vi "RT.vi"() -> ()   [LabVIEW 2014]
uses:
  support/Message Queue/Kapitza Message Queue.lvlib
  support/User Event - Stop/Kapitza User Event - Stop.lvlib
  support/Message Queue/Enqueue Message (Single).vi
  Classes/Abstract/Data/Data2D/Data2D.lvclass
  Classes/Abstract/Measurement/Measurement2D/Measurement2D.lvclass
  Classes/2D/RT/RT.lvclass
panel:
  in  "File Path Control":path=path "C:/Users/Sergei/Documents"
  in  "Driver 1":path=path "C:/Users/Sergei/YandexDisk/Лаборатория/Projects/Kapitza_prealpha/Drivers/Simulator.vi"
  in  "Driver 2":path=path "C:/Users/Sergei/YandexDisk/Лаборатория/Projects/Kapitza_prealpha/Drivers/Simulator.vi"
  in  "Address 2":refnum<visa-resource-name>
  in  "Address 1":refnum<visa-resource-name>
  in  "Stop":bool
  in  "Sample Name":string
  in  "Max":dbl
  in  "Step":dbl
  in  "Init":dbl
  in  "x0,5 step":bool
  out "y":dbl
  out "x":dbl
  in  "x2 step":bool
  in  "Start":bool
  out "XY Graph":cluster{"X":dbl[], "Y":dbl[]}[](graph)
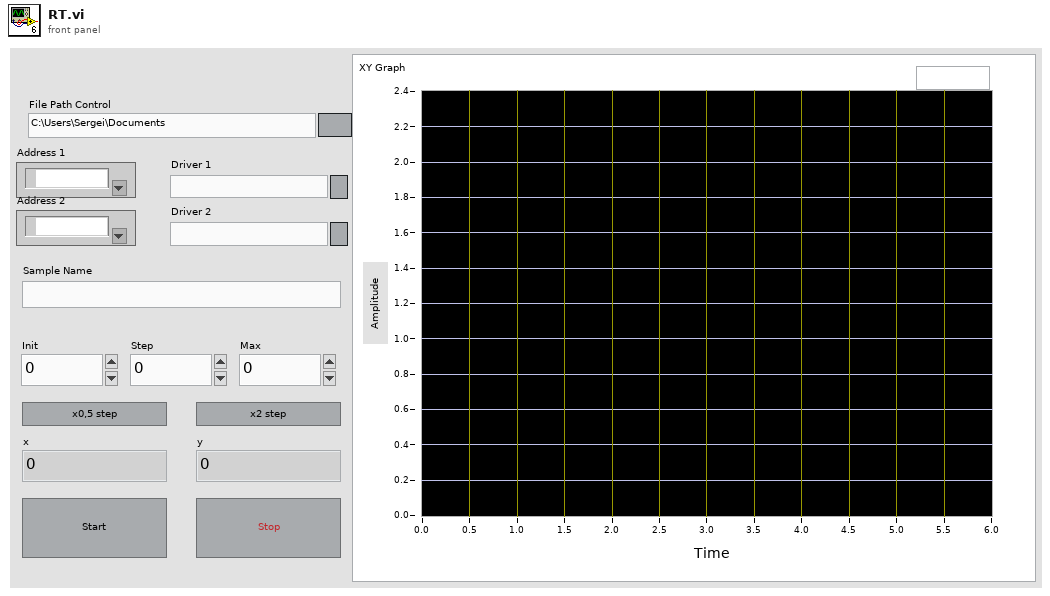
[diagram p1: front panel]
types:
  T1 = typedef "Kapitza Message Queue.lvlib/All Message Queues.ctl" = cluster{"UI":refnum<queue>}
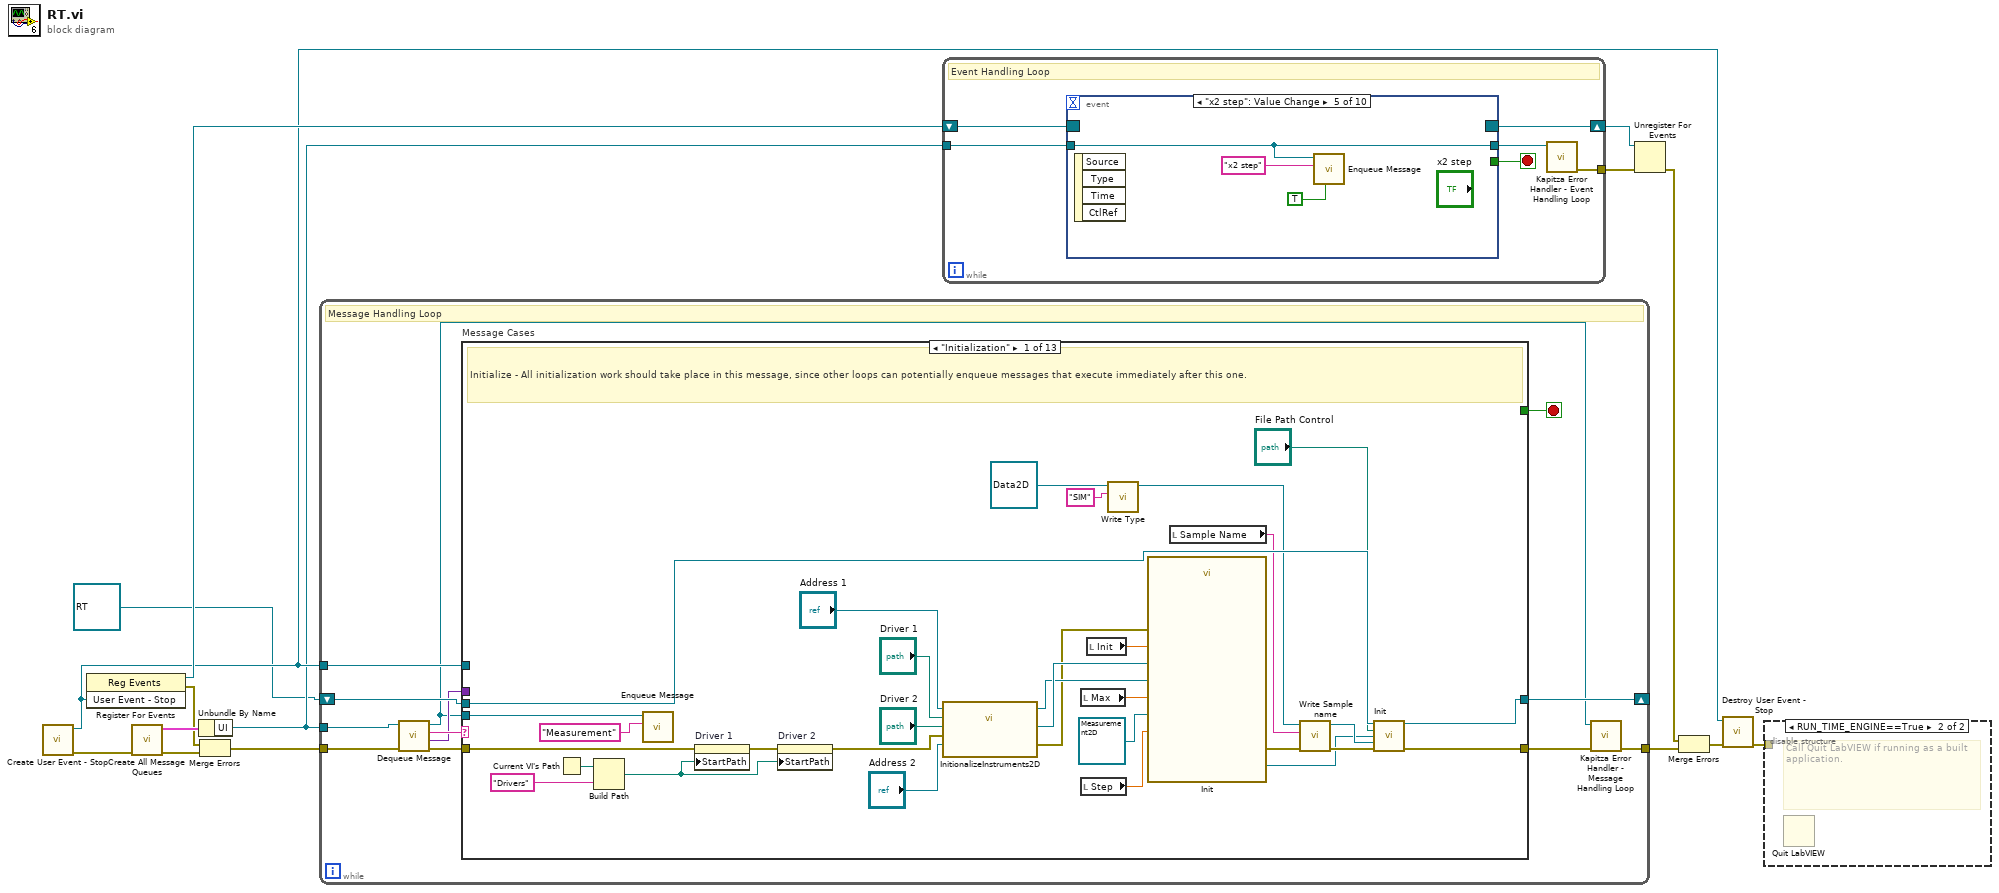
[diagram p0: block diagram]
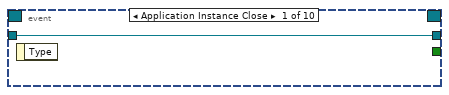
[diagram p3: hidden frame]
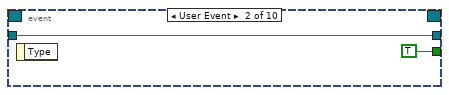
[diagram p4: hidden frame]
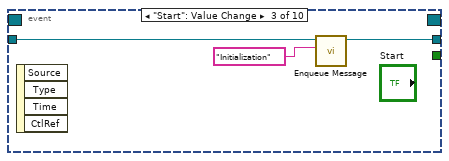
[diagram p5: hidden frame]
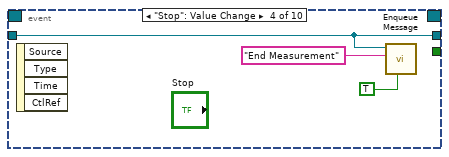
[diagram p6: hidden frame]
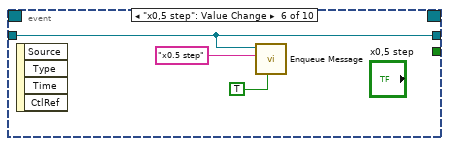
[diagram p7: hidden frame]
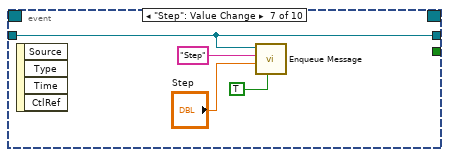
[diagram p8: hidden frame]
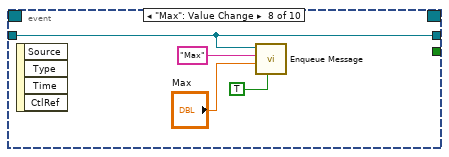
[diagram p9: hidden frame]
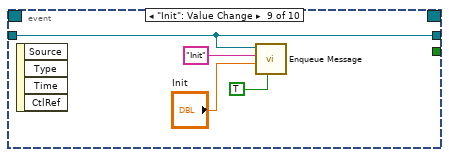
[diagram p10: hidden frame]
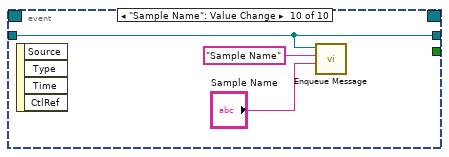
[diagram p11: hidden frame]
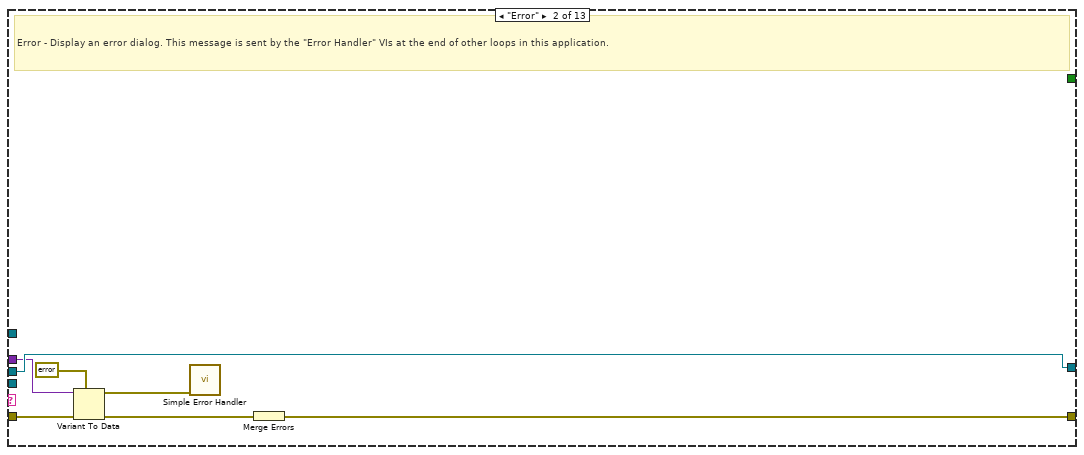
[diagram p12: hidden frame]
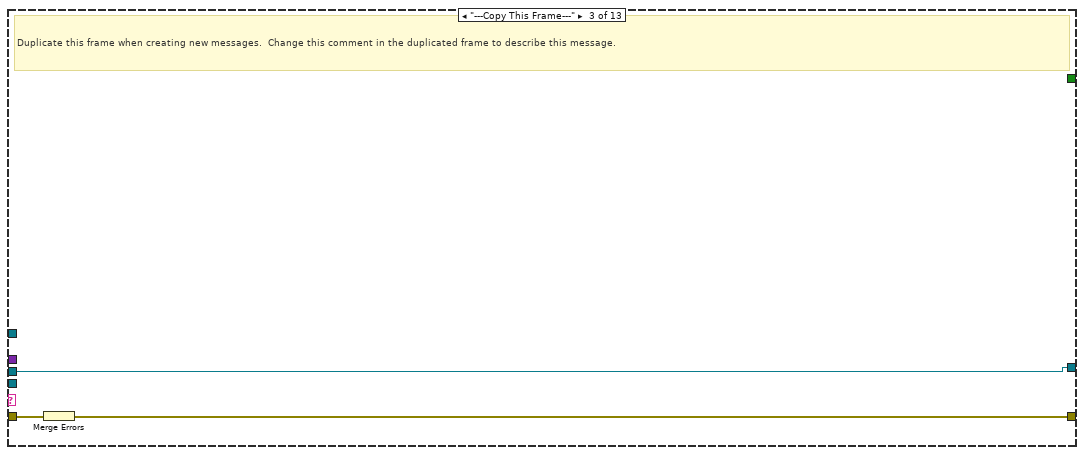
[diagram p13: hidden frame]
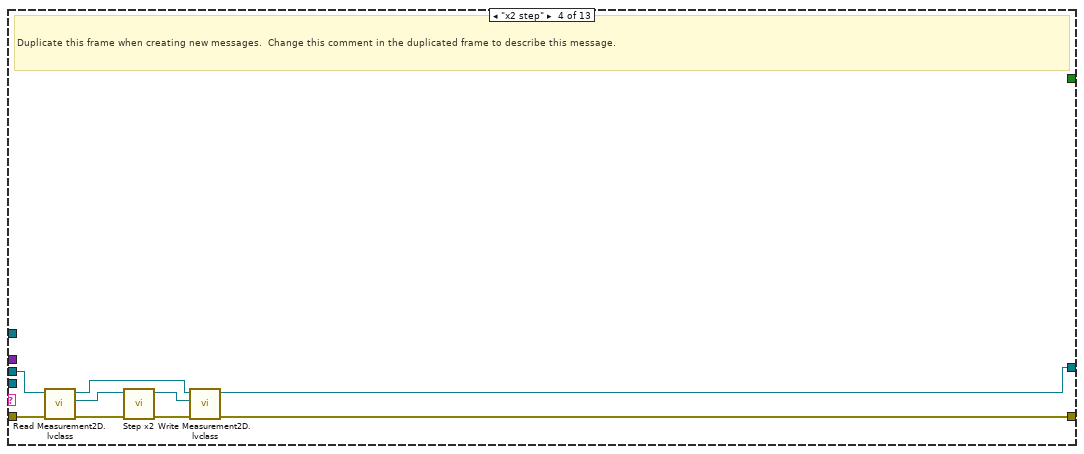
[diagram p14: hidden frame]
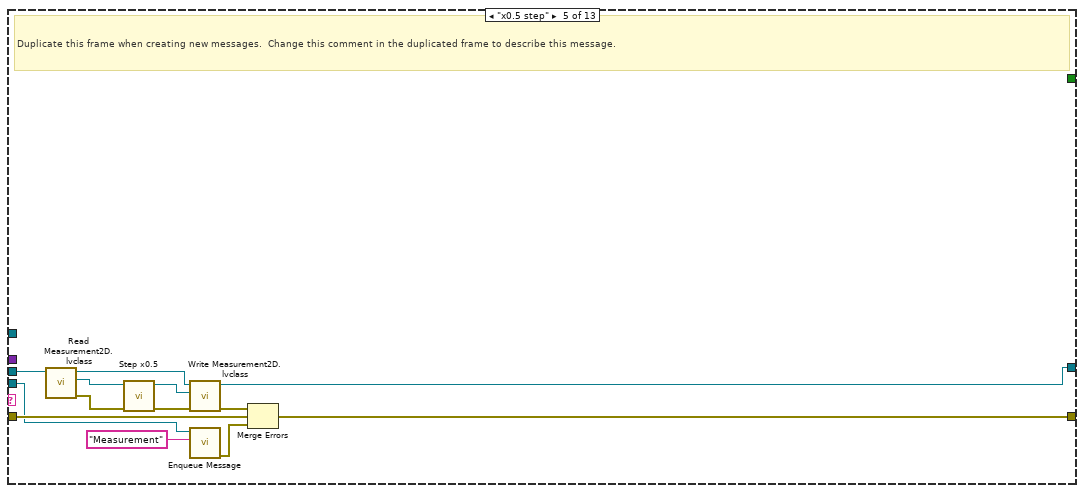
[diagram p15: hidden frame]
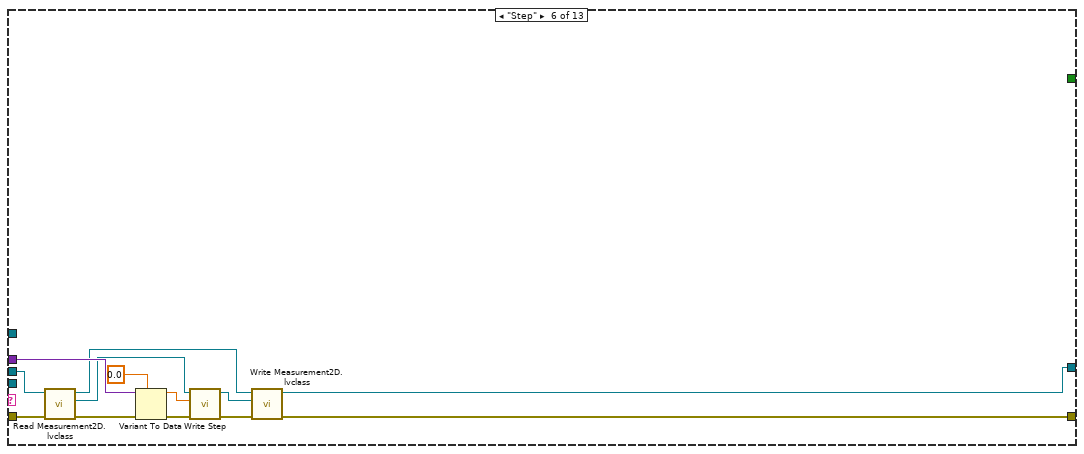
[diagram p16: hidden frame]
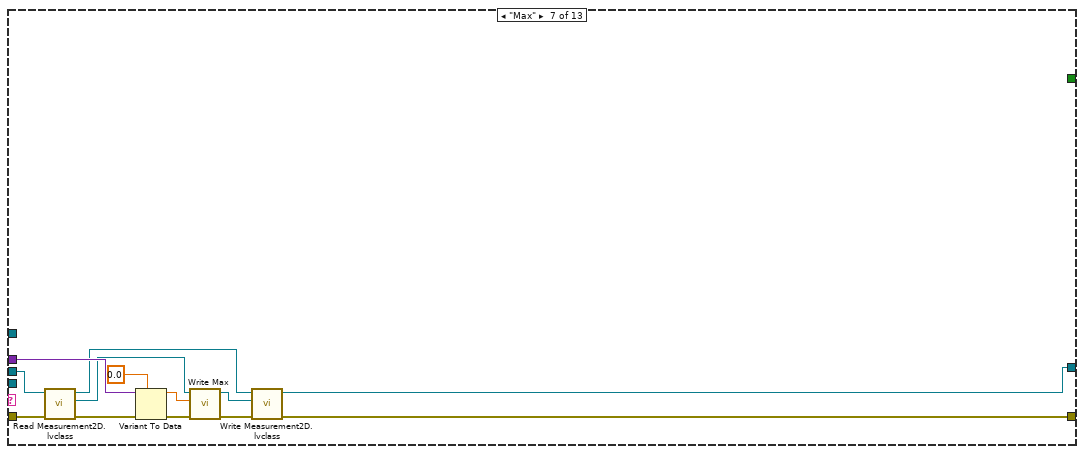
[diagram p17: hidden frame]
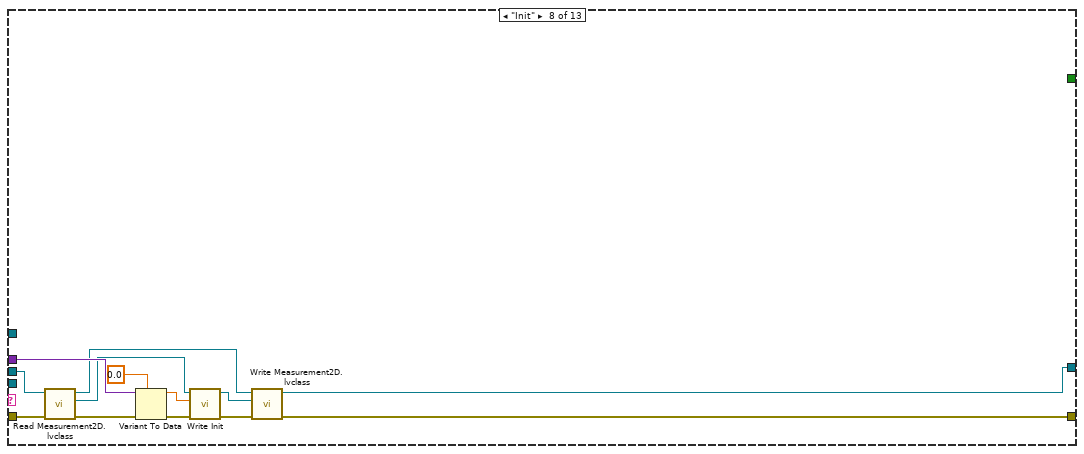
[diagram p18: hidden frame]
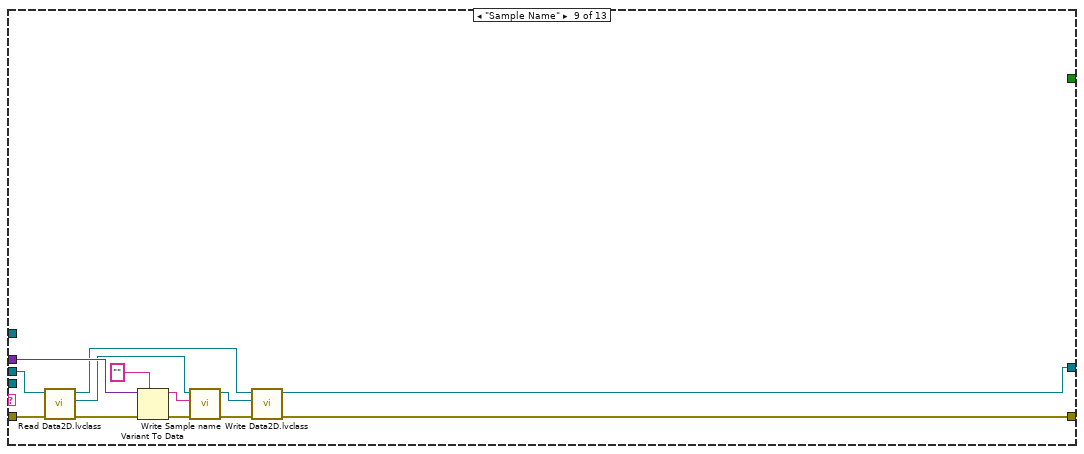
[diagram p19: hidden frame]
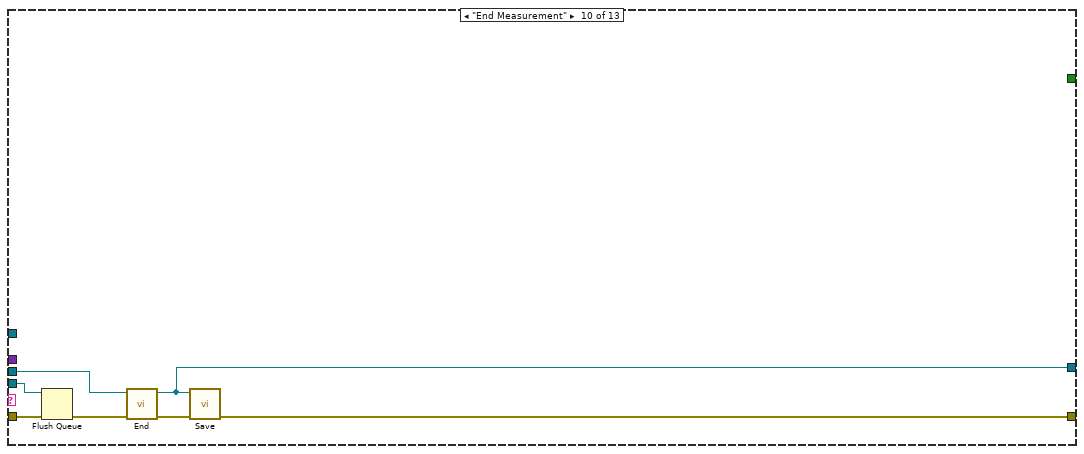
[diagram p20: hidden frame]
diagram:
  n1 = call "Create User Event - Stop.vi"() -> ("error out"=w13:errorcluster, "User Event - Stop"=w6:refnum<user-event>)  [unwired: 10 in]
  n2 = register-events(w6) -> (reference out=w7:refnum<event-registration>, error out=w4:errorcluster)  [unwired: 2 in]
  n3 = call "Create All Message Queues.vi"("error in (no error)"=w13) -> ("error out"=w2:errorcluster, "Message Queues out"=w15:T1)  [unwired: 9 in]
  n4 = Unbundle By Name(w15) -> ("UI"=w3:refnum<queue>)
  n5 = Merge Errors(w4, w2) -> (w5:errorcluster)
  n6 = while {
    tunnel: w3 -> [w19]
    shift-right: [w26] -> _
    shift-left: refnum<class "RT.lvclass"> refnum ("RT.lvclass") -> [w27]
    tunnel: w6 -> [w24]
    tunnel: w5 -> [w23]
    tunnel: [w17] -> w14
    stop <- w25 stop-if-true
    # "Message Handling Loop"
    n7 = call "Dequeue Message.vi"("error in (no error)"=w23, "Message Queue"=w19) -> ("error out"=w22:errorcluster, "Message Data"=w20:variant, "Message"=w21:string, "dup Message Queue"=w18:refnum<queue>)  [unwired: 6 in]
    n8 = case "Message Cases" shown="\"Initialization\"" w21 {
      tunnel: w18 -> [w33 _ _ _ w83 _ _ _ _ w147 w166 w187 _]
      tunnel: w22 -> [w38 w65 w68 w70 w90 w94 w108 w121 w134 w145 w151 w180 w188]
      tunnel: [w28 w59 w66 w69 w89 w91 w104 w117 w130 w143 w165 w183 w188] -> w16
      tunnel: w27 -> [w58 w64 w67 w77 w88 w100 w110 w126 w140 w149 w168 w186 w189]
      tunnel: [w57 w64 w67 w73 w86 w99 w109 w125 w139 w148 w157 w186 w189] -> w26
      tunnel: [_ _ _ _ _ _ _ _ _ _ _ TRUE _] -> w25
      tunnel: w20 -> [_ w63 _ _ _ w103 w116 w129 w142 _ _ w177 _]
      tunnel: w24 -> [_ _ _ _ _ _ _ _ _ _ _ w182 _]
      frame "Initialization" {
        # "Initialize - All initialization work should take place in this message, since other loops can potentially enqueue messages that execute immediately after this one."
        n9 = Current VI's Path() -> (path=w40:path)
        n10 = Build Path(base path=w40, name or relative path="Drivers") -> (appended path=w36:path)
        n11 = call-poly "Enqueue Message.vi"("Message"="Measurement", "Message Queue"=w33) -> ()  [unwired: 8 in, 2 out]
        n12 = property on="Driver 1" class="Path"(error in=w38, "StartPath"=w36) -> (error out=w37:errorcluster)  [unwired: 1 in, 1 out]
        n13 = property on="Driver 2" class="Path"(error in=w37, "StartPath"=w36) -> (error out=w35:errorcluster)  [unwired: 1 in, 1 out]
        n14 = call "InitionalizeInstruments2D.vi"("Address in"="Address 2", "error in (no error)"=w35, "Driver in"="Driver 2", "Driver 1"="Driver 1", "VISA Refnum in"="Address 1") -> ("error out"=w45:errorcluster, "Instrument out 2"=w52:refnum<class "Instrument.lvclass">, "Instrument out"=w51:refnum<class "Instrument.lvclass">)  [unwired: 4 in]
        n15 = local read "Max"() -> (w50:dbl)
        n16 = local read "Step"() -> (w49:dbl)
        n17 = local read "Init"() -> (w48:dbl)
        n18 = call-dynamic "Write Type.vi"("Type"="SIM", "Data2D in"=refnum<class "Data2D.lvclass"> refnum ("Data2D.lvclass")) -> ("Data2D out"=w30:refnum<class "Data2D.lvclass">)  [unwired: 8 in, 1 out]
        n19 = call-dynamic "Init.vi"("Instrument.lvclass 2"=w51, "Step"=w49, "Instrument 1.lvclass"=w52, "error in (no error)"=w45, "Max"=w50, "Init"=w48, "Measurement1D in"=refnum<class "Measurement2D.lvclass"> refnum) -> ("error out"=w44:errorcluster, "Measurement1D out"=w41:refnum<class "Measurement2D.lvclass">)  [unwired: 3 in]
        n20 = local read "Sample Name"() -> (w46:string)
        n21 = call-dynamic "Write Sample name.vi"("error in (no error)"=w44, "Sample name"=w46, "Data2D in"=w30) -> ("error out"=w43:errorcluster, "Data2D out"=w42:refnum<class "Data2D.lvclass">)  [unwired: 7 in]
        n22 = call-dynamic "Init.vi"("Experiment2D in"=w58, "Path"="File Path Control", "Measurement2D.lvclass"=w41, "Data2D.lvclass"=w42, "error in (no error)"=w43) -> ("Experiment2D out"=w57:refnum<class "RT.lvclass">, "error out"=w28:errorcluster)  [unwired: 9 in]
      }
      frame "Error" {
        # "Error - Display an error dialog. This message is sent by the \"Error Handler\" VIs at the end of other loops in this application."
        n23 = Variant To Data(error in=w65, type=errorcluster {"status"=FALSE, "code"=0, "source"=""} ("error constant"), Variant=w63) -> (data=w61:errorcluster, error out=w60:errorcluster)
        n24 = call <vilib>:"Simple Error Handler.vi"("error in (no error)"=w61) -> ()  [unwired: 4 in, 5 out]
        n25 = Merge Errors(w60) -> (w59:errorcluster)
      }
      frame "---Copy This Frame---" {
        # "Duplicate this frame when creating new messages.  Change this comment in the duplicated frame to describe this message."
        n26 = Merge Errors(w68) -> (w66:errorcluster)
      }
      frame "x2 step" {
        # "Duplicate this frame when creating new messages.  Change this comment in the duplicated frame to describe this message."
        n27 = call-dynamic "Read Measurement2D.lvclass.vi"("error in (no error)"=w70, "Experiment2D in"=w77) -> ("error out"=w72:errorcluster, "Measurement2D.lvclass"=w76:refnum<class "Measurement2D.lvclass">, "Experiment2D out"=w75:refnum<class "RT.lvclass">)  [unwired: 7 in]
        n28 = call-dynamic "Step x2.vi"("error in (no error)"=w72, "Measurement2D in"=w76) -> ("error out"=w71:errorcluster, "Measurement2D out"=w74:refnum<class "Measurement2D.lvclass">)  [unwired: 8 in]
        n29 = call-dynamic "Write Measurement2D.lvclass.vi"("error in (no error)"=w71, "Measurement2D.lvclass"=w74, "Experiment2D in"=w75) -> ("error out"=w69:errorcluster, "Experiment2D out"=w73:refnum<class "RT.lvclass">)  [unwired: 7 in]
      }
      frame "x0.5 step" {
        # "Duplicate this frame when creating new messages.  Change this comment in the duplicated frame to describe this message."
        n30 = call-dynamic "Read Measurement2D.lvclass.vi"("Experiment2D in"=w88) -> ("error out"=w78:errorcluster, "Measurement2D.lvclass"=w85:refnum<class "Measurement2D.lvclass">, "Experiment2D out"=w87:refnum<class "RT.lvclass">)  [unwired: 8 in]
        n31 = call-dynamic "Step x0.5.vi"("error in (no error)"=w78, "Measurement2D in"=w85) -> ("error out"=w79:errorcluster, "Measurement2D out"=w84:refnum<class "Measurement2D.lvclass">)  [unwired: 8 in]
        n32 = call-dynamic "Write Measurement2D.lvclass.vi"("error in (no error)"=w79, "Measurement2D.lvclass"=w84, "Experiment2D in"=w87) -> ("error out"=w81:errorcluster, "Experiment2D out"=w86:refnum<class "RT.lvclass">)  [unwired: 7 in]
        n33 = call-poly "Enqueue Message.vi"("Message"="Measurement", "Message Queue"=w83) -> ("error out"=w80:errorcluster)  [unwired: 8 in, 1 out]
        n34 = Merge Errors(w81, w90, w80) -> (w89:errorcluster)
      }
      frame "Step" {
        n35 = call-dynamic "Read Measurement2D.lvclass.vi"("error in (no error)"=w94, "Experiment2D in"=w100) -> ("error out"=w93:errorcluster, "Measurement2D.lvclass"=w98:refnum<class "Measurement2D.lvclass">, "Experiment2D out"=w101:refnum<class "RT.lvclass">)  [unwired: 7 in]
        n36 = Variant To Data(error in=w93, type=0.0, Variant=w103) -> (data=w97:dbl, error out=w92:errorcluster)
        n37 = call-dynamic "Write Step.vi"("error in (no error)"=w92, "Step"=w97, "Measurement2D in"=w98) -> ("error out"=w95:errorcluster, "Measurement2D out"=w96:refnum<class "Measurement2D.lvclass">)  [unwired: 7 in]
        n38 = call-dynamic "Write Measurement2D.lvclass.vi"("error in (no error)"=w95, "Measurement2D.lvclass"=w96, "Experiment2D in"=w101) -> ("error out"=w91:errorcluster, "Experiment2D out"=w99:refnum<class "RT.lvclass">)  [unwired: 7 in]
      }
      frame "Max" {
        n39 = call-dynamic "Read Measurement2D.lvclass.vi"("error in (no error)"=w108, "Experiment2D in"=w110) -> ("error out"=w107:errorcluster, "Measurement2D.lvclass"=w113:refnum<class "Measurement2D.lvclass">, "Experiment2D out"=w111:refnum<class "RT.lvclass">)  [unwired: 7 in]
        n40 = Variant To Data(error in=w107, type=0.0, Variant=w116) -> (data=w114:dbl, error out=w106:errorcluster)
        n41 = call-dynamic "Write Max.vi"("error in (no error)"=w106, "Max"=w114, "Measurement2D in"=w113) -> ("error out"=w105:errorcluster, "Measurement2D out"=w112:refnum<class "Measurement2D.lvclass">)  [unwired: 7 in]
        n42 = call-dynamic "Write Measurement2D.lvclass.vi"("error in (no error)"=w105, "Measurement2D.lvclass"=w112, "Experiment2D in"=w111) -> ("error out"=w104:errorcluster, "Experiment2D out"=w109:refnum<class "RT.lvclass">)  [unwired: 7 in]
      }
      frame "Init" {
        n43 = call-dynamic "Read Measurement2D.lvclass.vi"("error in (no error)"=w121, "Experiment2D in"=w126) -> ("error out"=w120:errorcluster, "Measurement2D.lvclass"=w124:refnum<class "Measurement2D.lvclass">, "Experiment2D out"=w127:refnum<class "RT.lvclass">)  [unwired: 7 in]
        n44 = Variant To Data(error in=w120, type=0.0, Variant=w129) -> (data=w123:dbl, error out=w119:errorcluster)
        n45 = call-dynamic "Write Init.vi"("error in (no error)"=w119, "Init"=w123, "Measurement2D in"=w124) -> ("error out"=w118:errorcluster, "Measurement2D out"=w122:refnum<class "Measurement2D.lvclass">)  [unwired: 7 in]
        n46 = call-dynamic "Write Measurement2D.lvclass.vi"("error in (no error)"=w118, "Measurement2D.lvclass"=w122, "Experiment2D in"=w127) -> ("error out"=w117:errorcluster, "Experiment2D out"=w125:refnum<class "RT.lvclass">)  [unwired: 7 in]
      }
      frame "Sample Name" {
        n47 = call-dynamic "Read Data2D.lvclass.vi"("error in (no error)"=w134, "Experiment2D in"=w140) -> ("error out"=w133:errorcluster, "Data2D.lvclass"=w137:refnum<class "Data2D.lvclass">, "Experiment2D out"=w135:refnum<class "RT.lvclass">)  [unwired: 7 in]
        n48 = Variant To Data(error in=w133, type="", Variant=w142) -> (data=w138:string, error out=w132:errorcluster)
        n49 = call-dynamic "Write Sample name.vi"("error in (no error)"=w132, "Sample name"=w138, "Data2D in"=w137) -> ("error out"=w131:errorcluster, "Data2D out"=w136:refnum<class "Data2D.lvclass">)  [unwired: 7 in]
        n50 = call-dynamic "Write Data2D.lvclass.vi"("error in (no error)"=w131, "Data2D.lvclass"=w136, "Experiment2D in"=w135) -> ("error out"=w130:errorcluster, "Experiment2D out"=w139:refnum<class "RT.lvclass">)  [unwired: 7 in]
      }
      frame "End Measurement" {
        n51 = Flush Queue(queue=w147, error in (no error)=w145) -> (error out=w144:errorcluster)  [unwired: 2 out]
        n52 = call-dynamic "End.vi"("error in (no error)"=w144, "Experiment2D in"=w149) -> ("error out"=w146:errorcluster, "Experiment2D out"=w148:refnum<class "RT.lvclass">)  [unwired: 8 in]
        n53 = call-dynamic "Save.vi"("error in (no error)"=w146, "Experiment2D in"=w148) -> ("error out"=w143:errorcluster)  [unwired: 8 in, 1 out]
      }
      frame "Measurement" {
        # "Duplicate this frame when creating new messages.  Change this comment in the duplicated frame to describe this message."
        n54 = call-dynamic "Measurement.vi"("error in (no error)"=w151, "Experiment2D in"=w168) -> ("error out"=w152:errorcluster, "Finish?"=w167:bool, "Experiment2D out"=w164:refnum<class "RT.lvclass">)  [unwired: 6 in, 1 out]
        n55 = Wait (ms)(milliseconds to wait=u32 100) -> ()  [unwired: 1 out]
        n56 = call-dynamic "Graph.vi"("error in (no error)"=w152, "Experiment2D in"=w164) -> ("error out"=w153:errorcluster, "Y"=w158:dbl[], "X"=w159:dbl[], "Experiment2D out"=w157:refnum<class "RT.lvclass">)  [unwired: 6 in]
        n57 = call-dynamic "Get point.vi"("error in (no error)"=w153, "Experiment2D in"=w157) -> ("error out"=w154:errorcluster, "y"=→"y":dbl, "x"=→"x":dbl)  [unwired: 6 in, 1 out]
        n58 = call "Convert to Dynamic Data"("Array"=w159) -> ("Dynamic Data Type"=w162:dynamicdata)  [unwired: 3 in]
        n59 = call "Convert to Dynamic Data2"("Array"=w158) -> ("Dynamic Data Type"=w161:dynamicdata)  [unwired: 3 in]
        n60 = call "Build XY Graph"("error in (no error)"=w154, "Y Input"=w161, "X Input"=w162) -> ("error out"=w150:errorcluster, "XY Graph"=→"XY Graph":cluster{"X":dbl[], "Y":dbl[]}[])  [unwired: 7 in]
        n61 = case shown="False" w167 {
          tunnel: w166 -> [w171 w176]
          tunnel: w150 -> [w170 w174]
          tunnel: [w169 w173] -> w165
          frame False {
            n62 = call-poly "Enqueue Message.vi"("error in (no error)"=w170, "Message"="Measurement", "Message Queue"=w171) -> ("error out"=w169:errorcluster)  [unwired: 7 in, 1 out]
          }
          frame True {
            n63 = call-poly "Enqueue Message.vi"("error in (no error)"=w174, "Message"="End Measurement", "Message Queue"=w176) -> ("error out"=w173:errorcluster)  [unwired: 7 in, 1 out]
          }
        }
      }
      frame "Exit" {
        # "Exit - Exit the application."
        n64 = Release Queue(queue=w187, error in (no error)=w180) -> (error out=w184:errorcluster)  [unwired: 1 in, 2 out]
        n65 = call "Fire User Event - Stop.vi"("User Event - Stop"=w182) -> ("error out"=w181:errorcluster)  [unwired: 10 in]
        n66 = Variant To Data(type=errorcluster {"status"=FALSE, "code"=0, "source"=""} ("error constant"), Variant=w177) -> (data=w178:errorcluster)  [unwired: 1 in, 1 out]
        n67 = Merge Errors(w181, w184) -> (w183:errorcluster)
        n68 = call <vilib>:"Simple Error Handler.vi"("error in (no error)"=w178) -> ()  [unwired: 4 in, 5 out]
      }
      frame Default {
        # "'Default' case only runs if there is a message that isn't defined in any of the other cases"
      }
    }
    n69 = call "Kapitza Error Handler - Message Handling Loop.vi"("error in (no error)"=w16, "Message Queue"=w18) -> ("dup error in"=w17:errorcluster)  [unwired: 8 in, 1 out]
  }
  n70 = while {
    tunnel: w3 -> [w195]
    shift-right: [w193] -> w10
    shift-left: w7 -> [w194]
    tunnel: [w190] -> w8
    stop <- w192 stop-if-true
    # "Event Handling Loop"
    n71 = event shown="[4] \"x2 step\": Value Change" {
      selector: w194 -> [_ _ _ _ _ _ _ _ _ _]
      dyn-events: [_ _ _ _ _ _ _ _ _ _] -> w193
      timeout: _ -> [_ _ _ _ _ _ _ _ _ _]
      tunnel: [_ TRUE ("Discard?") _ _ _ _ _ _ _ _] -> w192
      tunnel: w195 -> [w196 w198 w201 w204 w207 w208 w213 w216 w220 w224]
      tunnel: [w196 w198 w200 w204 w207 w208 w213 w216 w220 w224] -> w191
      event Application Instance Close {
        n72 = event-data() -> ()  [unwired: 1 in, 1 out]
      }
      event User Event {
        n73 = event-data() -> ()  [unwired: 1 in, 1 out]
      }
      event "Start": Value Change {
        n74 = event-data() -> ()  [unwired: 1 in, 4 out]
        n75 = call-poly "Enqueue Message.vi"("Message"="Initialization", "Message Queue"=w201) -> ("dup Message Queue"=w200:refnum<queue>)  [unwired: 8 in, 1 out]
      }
      event "Stop": Value Change {
        n76 = event-data() -> ()  [unwired: 1 in, 4 out]
        n77 = call-poly "Enqueue Message.vi"("Priority Message? (F)"=TRUE, "Message"="End Measurement", "Message Queue"=w204) -> ()  [unwired: 7 in, 2 out]
      }
      event "x2 step": Value Change {
        n78 = event-data() -> ()  [unwired: 1 in, 4 out]
        n79 = call-poly "Enqueue Message.vi"("Priority Message? (F)"=TRUE, "Message"="x2 step", "Message Queue"=w207) -> ()  [unwired: 7 in, 2 out]
      }
      event "x0,5 step": Value Change {
        n80 = event-data() -> ()  [unwired: 1 in, 4 out]
        n81 = call-poly "Enqueue Message.vi"("Priority Message? (F)"=TRUE, "Message"="x0.5 step", "Message Queue"=w208) -> ()  [unwired: 7 in, 2 out]
      }
      event "Step": Value Change {
        n82 = event-data() -> ()  [unwired: 1 in, 4 out]
        n83 = call-poly "Enqueue Message.vi"("Priority Message? (F)"=TRUE, "Message Data"="Step", "Message"="Step", "Message Queue"=w213) -> ()  [unwired: 6 in, 2 out]
      }
      event "Max": Value Change {
        n84 = event-data() -> ()  [unwired: 1 in, 4 out]
        n85 = call-poly "Enqueue Message.vi"("Priority Message? (F)"=TRUE, "Message Data"="Max", "Message"="Max", "Message Queue"=w216) -> ()  [unwired: 6 in, 2 out]
      }
      event "Init": Value Change {
        n86 = event-data() -> ()  [unwired: 1 in, 4 out]
        n87 = call-poly "Enqueue Message.vi"("Priority Message? (F)"=TRUE, "Message Data"="Init", "Message"="Init", "Message Queue"=w220) -> ()  [unwired: 6 in, 2 out]
      }
      event "Sample Name": Value Change {
        n88 = event-data() -> ()  [unwired: 1 in, 4 out]
        n89 = call-poly "Enqueue Message.vi"("Message Data"="Sample Name", "Message"="Sample Name", "Message Queue"=w224) -> ()  [unwired: 7 in, 2 out]
      }
    }
    n90 = call "Kapitza Error Handler - Event Handling Loop.vi"("Message Queue"=w191) -> ("dup error in"=w190:errorcluster)  [unwired: 9 in, 1 out]
  }
  n91 = Unregister For Events(event registration refnum=w10, error in=w8) -> (error out=w11:errorcluster)
  n92 = Merge Errors(w11, w14) -> (w12:errorcluster)
  n93 = call "Destroy User Event - Stop.vi"("error in (no error)"=w12, "User Event - Stop"=w6) -> ("error out"=w9:errorcluster)  [unwired: 9 in]
  n94 = disable-structure shown="RUN_TIME_ENGINE==True" {
    disable-tunnel: w9 -> [_ _]
    frame condition #0 (active) {
    }
    frame condition #1 {
      # "Call Quit LabVIEW if running as a built application."
      n95 = Quit LabVIEW() -> ()  [unwired: 1 in]
    }
  }
